vi "Fit VI window to Largest Dec__ogtk.vi"(4 "error in (no error)":errorcluster, 6 "border spacing (2 px)":i32=2, 7 "VI Ref (calling VI)":refnum<vi>) -> (0 "error out":errorcluster, 3 "dup VI Ref":refnum<vi>)   [LabVIEW 2011]
doc: "This utility will fit (resize and center) a VI (defined by the \"VI Ref\" input) about the largest decoration in that VI. It will add a border defined by border spacing in units of pixels. If there are no decorations found in the VI it is a no-op and will not produce an error. Unfortunately, this VI can not find locked decorations (yet)."
panel:
  # "Fit VI window to Largest Decoration.vi\n\nFits a VI's front panel window to its largest decoration size.\n\nPlease visit http://www.OpenG.org to learn about the\nOpen Source LabVIEW software movement.\n\nNOTICE -- YOU MUST LEAVE THIS NOTICE IN PLACE.  PER THE TERMS OF THE LICENSE BELOW, YOU MAY SUBLICENSE THIS SOFTWARE \nIN ANY WAY THAT DOES NOT CONFLICT WITH THIS LICENSE.\n\n### BSD License (http://www.opensource.org/licenses/bsd-license.php) Begin ###\n \nCopyright (c) 2002, Jim Kring <jim@jimkring.com>\nCopyright (c) 2002, Cal-Bay Systems, Inc. <info@calbay.com>\n\nAll rights reserved.\n\nRedistribution and use in source and binary forms, with or without modification, are permitted provided that the following conditions are met:\n\n    * Redistributions of source code must retain the above copyright notice, this list of conditions and the following disclaimer.\n    * Redistributions in binary form must reproduce the above copyright notice, this list of conditions and the following disclaimer in the \n       documentation and/or other materials provided with the distribution.\n    * Neither the name of SciWare, James Kring, Inc., nor the names of its contributors may be used to endorse or promote products derived \n       from this software without specific prior written permission.\n\nTHIS SOFTWARE IS PROVIDED BY THE COPYRIGHT HOLDERS AND CONTRIBUTORS \"AS IS\" AND ANY EXPRESS OR IMPLIED WARRANTIES, \nINCLUDING, BUT NOT LIMITED TO, THE IMPLIED WARRANTIES OF MERCHANTABILITY AND FITNESS FOR A PARTICULAR PURPOSE ARE \nDISCLAIMED. IN NO EVENT SHALL THE COPYRIGHT OWNER OR CONTRIBUTORS BE LIABLE FOR ANY DIRECT, INDIRECT, INCIDENTAL,\n SPECIAL, EXEMPLARY, OR CONSEQUENTIAL DAMAGES (INCLUDING, BUT NOT LIMITED TO, PROCUREMENT OF SUBSTITUTE GOODS OR \nSERVICES; LOSS OF USE, DATA, OR PROFITS; OR BUSINESS INTERRUPTION) HOWEVER CAUSED AND ON ANY THEORY OF LIABILITY, \nWHETHER IN CONTRACT, STRICT LIABILITY, OR TORT (INCLUDING NEGLIGENCE OR OTHERWISE) ARISING IN ANY WAY OUT OF THE USE \nOF THIS SOFTWARE, EVEN IF ADVISED OF THE POSSIBILITY OF SUCH DAMAGE.\n\n### BSD License End ###"
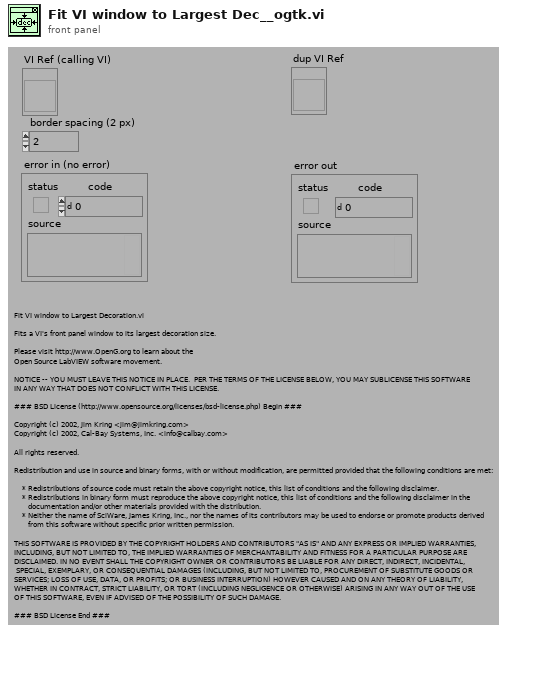
[diagram p1: front panel]
types:
  T1 = typedef "LVRectTypeDef.ctl" = cluster{"left":i16, "top":i16, "right":i16, "bottom":i16}
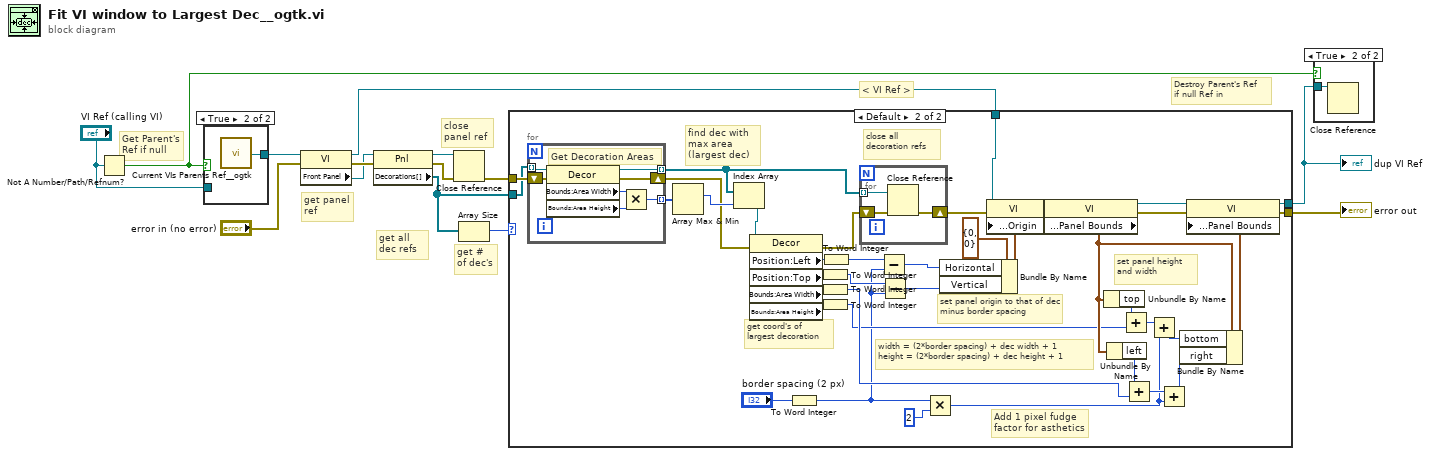
[diagram p0: block diagram]
diagram:
  # "Destroy Parent's Ref\nif null Ref in"
  # "Get Parent's\nRef if null"
  # "get # of dec's"
  # "get panel ref"
  # "get all dec refs"
  # "close panel ref"
  # "< VI Ref >"
  n1 = Not A Number/Path/Refnum?(number/path/refnum="VI Ref (calling VI)") -> (NaN/Path/Refnum?=w2:bool)
  n2 = case shown="True" w2 {
    tunnel: [w15 w16] -> w3
    tunnel: "VI Ref (calling VI)" -> [w15 _]
    frame False {
    }
    frame True {
      n3 = call "Current VIs Parents Ref__ogtk.vi"() -> ("Calling VI's Reference"=w16:refnum<vi>)  [unwired: 2 in]
    }
  }
  n4 = property on="Property Node" class="VI"(reference=w3, error in="error in (no error)") -> (reference out=w14:refnum<vi>, error out=w12:errorcluster, "Front Panel"=w9:refnum<vi>)
  n5 = property on="Property Node" class="Pnl"(reference=w9, error in=w12) -> (reference out=w13:refnum<vi>, error out=w11:errorcluster, "Decorations[]"=w6:refnum<vi>[])
  n6 = Close Reference(reference=w13, error in (no error)=w11) -> (error out=w8:errorcluster)
  n7 = Array Size(array=w6) -> (size(s)=w5:i32)
  n8 = case shown="Default" w5 {
    tunnel: w14 -> [w18 w56]
    tunnel: w8 -> [w17 w39]
    tunnel: [w17 w27] -> w7
    tunnel: [w18 w26] -> w1
    tunnel: w6 -> [_ w25]
    frame 0 {
      # "do nothing if no decorations"
    }
    frame Default {
      # "width = (2*border spacing) + dec width + 1\nheight = (2*border spacing) + dec height + 1"
      # "set panel height and width"
      # "set panel origin to that of dec minus border spacing"
      # "close all  decoration refs"
      # "get coord's of largest decoration"
      # "Add 1 pixel fudge factor for asthetics"
      # "find dec with max area (largest dec)"
      n9 = for {
        tunnel: w25 -> [w65] mode=indexing
        tunnel: [w62] -> w38 mode=indexing
        shift-right: [w60] -> w34
        shift-left: w39 -> [w61]
        tunnel: [w59] -> w36 mode=indexing
        # "Get Decoration Areas"
        n10 = property class="Decor"(reference=w65, error in=w61) -> (reference out=w59:refnum<vi>, error out=w60:errorcluster, "Bounds:Area Width"=w64:u32, "Bounds:Area Height"=w63:u32)
        n11 = Multiply(x=w64, y=w63) -> (x*y=w62:u32)
      }
      n12 = Array Max & Min(array=w38) -> (max index (indices)=w37:i32)  [unwired: 3 out]
      n13 = Index Array(array=w36, index=w37) -> (element=w35:refnum<vi>)
      n14 = property class="Decor"(reference=w35, error in=w34) -> (error out=w33:errorcluster, "Position:Left"=w42:i32, "Position:Top"=w45:i32, "Bounds:Area Width"=w50:u32, "Bounds:Area Height"=w48:u32)  [unwired: 1 out]
      n15 = To Word Integer(number="border spacing (2 px)") -> (16bit integer=w19:i16)
      n16 = To Word Integer(number=w45) -> (16bit integer=w20:i16)
      n17 = To Word Integer(number=w50) -> (16bit integer=w23:i16)
      n18 = To Word Integer(number=w48) -> (16bit integer=w22:i16)
      n19 = To Word Integer(number=w42) -> (16bit integer=w21:i16)
      n20 = for {
        tunnel: w36 -> [w68] mode=indexing
        shift-right: [w66] -> w30
        shift-left: w33 -> [w67]
        n21 = Close Reference(reference=w68, error in (no error)=w67) -> (error out=w66:errorcluster)
      }
      n22 = Subtract(x=w21, y=w19) -> (x-y=w43:i16)
      n23 = Subtract(x=w20, y=w19) -> (x-y=w44:i16)
      n24 = Multiply(x=w19, y=i16 2) -> (x*y=w24:i16)
      n25 = Bundle By Name(cluster=cluster{"Horizontal":i16, "Vertical":i16} {"Horizontal"=0, "Vertical"=0} ("Front Panel Window:Origin"), "Horizontal"=w43, "Vertical"=w44) -> (w40:cluster{"Horizontal":i16, "Vertical":i16})
      n26 = property on="Property Node" class="VI"(reference=w56, error in=w30, "Front Panel Window:Origin"=w40) -> (reference out=w57:refnum<vi>, error out=w29:errorcluster)
      n27 = property on="Property Node" class="VI"(reference=w57, error in=w29) -> (reference out=w58:refnum<vi>, error out=w28:errorcluster, "Front Panel Window:Panel Bounds"=w46:T1)
      n28 = Unbundle By Name(w46) -> ("top"=w47:i16)
      n29 = Unbundle By Name(w46) -> ("left"=w49:i16)
      n30 = Add(x=w47, y=w22) -> (x+y=w54:i16)
      n31 = Add(x=w49, y=w23) -> (x+y=w52:i16)
      n32 = Add(x=w54, y=w24) -> (x+y=w55:i16)
      n33 = Add(x=w52, y=w24) -> (x+y=w53:i16)
      n34 = Bundle By Name(cluster=w46, "bottom"=w55, "right"=w53) -> (w51:T1)
      n35 = property on="Property Node" class="VI"(reference=w58, error in=w28, "Front Panel Window:Panel Bounds"=w51) -> (reference out=w26:refnum<vi>, error out=w27:errorcluster)
    }
  }
  "error out" <- w7
  "dup VI Ref" <- w1
  n36 = case shown="True" w2 {
    tunnel: w1 -> [_ w69]
    frame False {
    }
    frame True {
      n37 = Close Reference(reference=w69) -> ()  [unwired: 1 in, 1 out]
    }
  }
